vi "ROSSubscriber.vi"(2 "Response":T2, 3 "ROS":T3={"topic port"=1236, "Node"="/labview", "topic"="/robot/head/command_head_nod", "type"="std_msgs/Bool", "node port"=7000, "error "={"status"=FALSE, "code"=0, "source"=""}, "Direction"=enum."Publisher", "Update (ms)"=1, "FIFO size"=1}) -> ()   [LabVIEW 2012]
doc: "Lists nodes with a given topic, requests topics, opens new ports for sunscribers, updates subscribers with master, and closes subscribers"
uses:
  _ROSDefinition.vi
  SubVIs/_ROSDirection.ctl
  SubVIs/_ROSControl.ctl
panel:
  out "publishers":T1(array[cluster])
  out "Queue log":string
  out "read":string
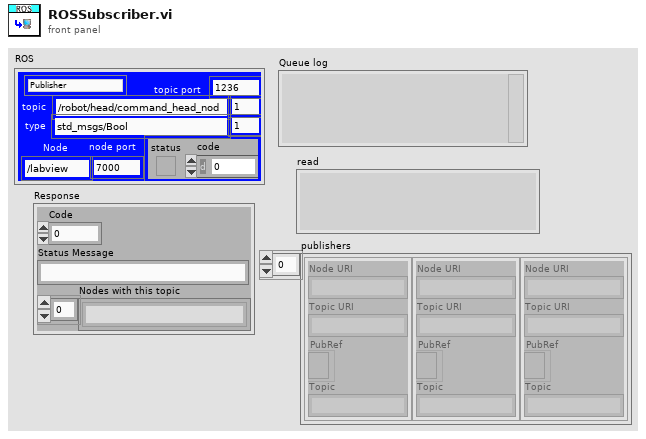
[diagram p1: front panel]
types:
  T1 = cluster{"Node URI":string, "Topic URI":string, "PubRef":refnum<k5>, "Topic":string}[]
  T2 = cluster{"Code":i32, "Status Message":string, "Nodes with this topic":string[]}
  T3 = typedef "_ROSControl.ctl" = cluster{"topic port":u16, "Node":string, "topic":string, "type":string, "node port":u16, "error ":errorcluster, "Direction":T4, "Update (ms)":u16, "FIFO size":u16}
  T4 = typedef "_ROSDirection.ctl" = enum16{"Node", "Publisher", "Subscriber", "ServiceClient", "ServiceProvider"}
  T5 = enum16{"Reset Log", "Add Client", "Remove Client", "Add Task"}
  T6 = cluster{"Node URI":string, "Topic URI":string, "PubRef":refnum<k5>, "Topic":string}
  T7 = cluster{"Caller ID":string, "Topic Name":string, "Node URIs":string[]}
  T8 = cluster{"Protocol":string, "Code":i32, "IP":string, "Port":i32}
  T9 = cluster{"Protocol":string, "Topic URI":string, "PubRef":refnum<k5>, "topic":string}
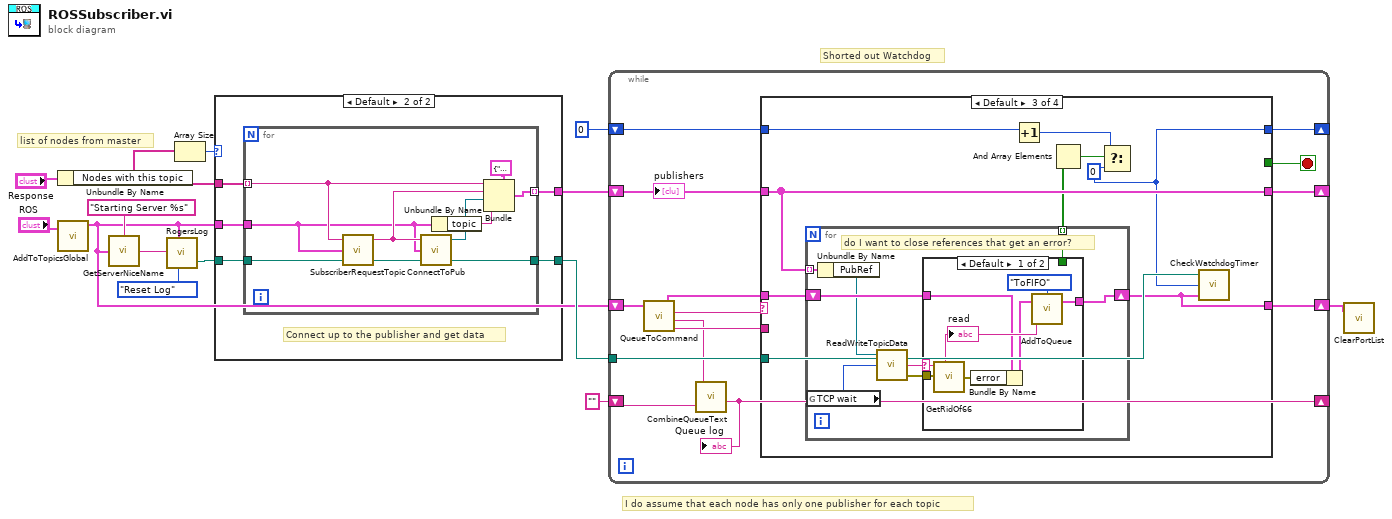
[diagram p0: block diagram]
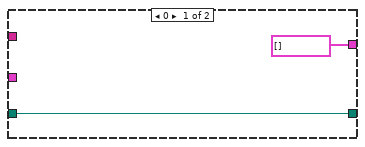
[diagram p2: hidden frame]
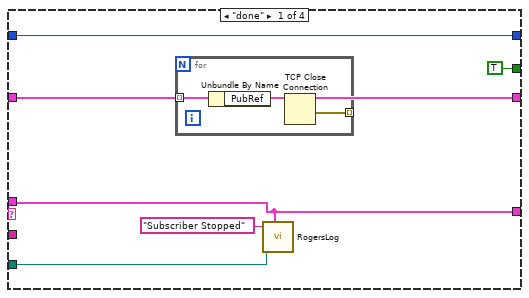
[diagram p3: hidden frame]
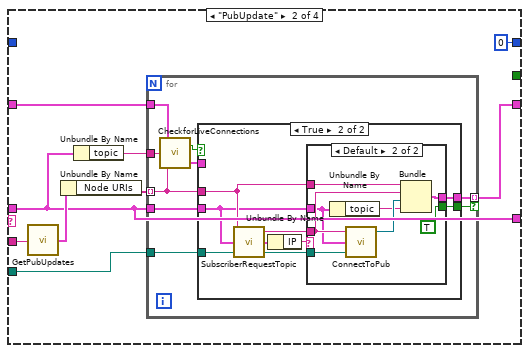
[diagram p4: hidden frame]
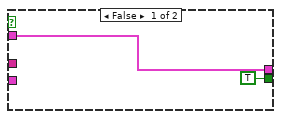
[diagram p5: hidden frame]
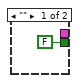
[diagram p6: hidden frame]
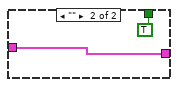
[diagram p7: hidden frame]
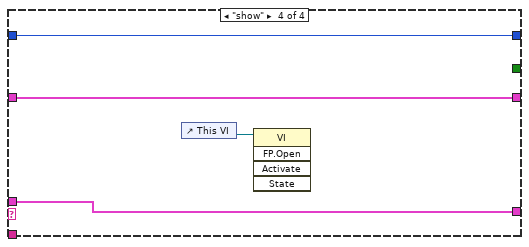
[diagram p8: hidden frame]
diagram:
  # "Shorted out Watchdog"
  # "I do assume that each node has only one publisher for each topic"
  # "list of nodes from master"
  n1 = Unbundle By Name("Response") -> ("Nodes with this topic"=w6:string[])
  n2 = call "AddToTopicsGlobal.vi"("ROS in"="ROS") -> ("ROS out"=w1:T3)  [unwired: 2 in]
  n3 = call "GetServerNiceName.vi"("ROS"=w1, "Text to add"="Starting Server %s") -> ("String"=w11:string)
  n4 = call "RogersLog.vi"("Text to add"=w11, "ROS"=w1, "Task"=T5."Reset Log") -> ("LogPath out"=w9:path)  [unwired: 2 in, 1 out]
  n5 = Array Size(array=w6) -> (size(s)=w5:i32)
  n6 = case shown="Default" w5 {
    tunnel: w6 -> [_ w21]
    tunnel: [T1 [] w20] -> w13
    tunnel: w9 -> [w15 w19]
    tunnel: w1 -> [_ w18]
    tunnel: [w15 w17] -> w8
    frame 0 {
    }
    frame Default {
      # "Connect up to the publisher and get data"
      n7 = for {
        tunnel: w21 -> [w28] mode=indexing
        tunnel: [w25] -> w20 mode=indexing
        tunnel: w19 -> [w31]
        tunnel: w18 -> [w23]
        tunnel: [w29] -> w17
        n8 = call "SubscriberRequestTopic.vi"("LogPath in"=w31, "ROS"=w23, "Node URI"=w28) -> ("LogPath out"=w30:path, "Topic URI"=w27:string)  [unwired: 1 out]
        n9 = call "ConnectToPub.vi"("LogPath in"=w30, "ROS"=w23, "IP"=w27) -> ("LogPath out"=w29:path, "PubRef"=w26:refnum<k5>)  [unwired: 1 out]
        n10 = Unbundle By Name(w23) -> ("topic"=w22:string)
        n11 = Bundle(cluster=T6 {"Node URI"="", "Topic URI"="", "PubRef"=refnum, "Topic"=""} ("output cluster"), "Node URI"=w28, "Topic URI"=w27, "PubRef"=w26, "Topic"=w22) -> (w25:T6)
      }
    }
  }
  n12 = while {
    shift-right: [w41] -> _
    shift-left: w13 -> [w45]
    tunnel: w8 -> [w40]
    shift-right: [w38] -> _
    shift-left: 0 -> [w39]
    shift-right: [w35] -> _
    shift-left: "" ("New List") -> [w37]
    shift-right: [w32] -> w3
    shift-left: w1 -> [w34]
    stop <- w43 stop-if-true
    n13 = call "QueueToCommand.vi"("ROS"=w34) -> ("ROS out"=w33:T3, "Command"=w44:string, "Queue log"=w36:string, "data"=w42:string)  [unwired: 2 in]
    n14 = call "CombineQueueText.vi"("Old List"=w37, "Queue In"=w36) -> ("New List"=w35:string)  [unwired: 1 in]
    "Queue log" <- w35
    n15 = case shown="Default" w44 {
      tunnel: w45 -> [w50 w57 w101 w122]
      tunnel: [TRUE _ _ _] -> w43
      tunnel: w42 -> [_ w61 _ _]
      tunnel: [w50 w58 w101 w122] -> w41
      tunnel: w33 -> [w46 w55 w94 w119]
      tunnel: w40 -> [w48 w59 w96 _]
      tunnel: w39 -> [w47 _ w97 w120]
      tunnel: [w47 0 w95 w120] -> w38
      tunnel: [w46 w55 w93 w119] -> w32
      frame "done" {
        n16 = for {
          tunnel: w50 -> [w53] mode=indexing
          tunnel: [w54] -> _ mode=indexing
          n17 = Unbundle By Name(w53) -> ("PubRef"=w52:refnum<k5>)
          n18 = TCP Close Connection(connection ID=w52) -> (error out=w54:errorcluster)  [unwired: 2 in, 1 out]
        }
        n19 = call "RogersLog.vi"("Text to add"="Subscriber Stopped", "ROS"=w46, "LogPath in"=w48) -> ()  [unwired: 2 in, 2 out]
      }
      frame "PubUpdate" {
        n20 = call "GetPubUpdates.vi"("XML"=w61) -> ("PubUpdate"=w62:T7)
        n21 = Unbundle By Name(w62) -> ("Node URIs"=w60:string[])
        n22 = Unbundle By Name(w55) -> ("topic"=w56:string)
        n23 = for {
          tunnel: w60 -> [w68] mode=indexing
          tunnel: w59 -> [w72]
          tunnel: w55 -> [w71]
          tunnel: [w70] -> w58 mode=indexing if=w64
          tunnel: w57 -> [w69]
          tunnel: w56 -> [w65]
          n24 = call "CheckforLiveConnections.vi"("Node URI"=w68, "topic"=w65, "Connections"=w69) -> ("Connection"=w66:T6, "new?"=w67:bool)
          n25 = case shown="True" w67 {
            tunnel: w72 -> [_ w83]
            tunnel: w71 -> [_ w78]
            tunnel: w68 -> [_ w81]
            tunnel: [w74 w79] -> w70
            tunnel: w66 -> [w74 _]
            tunnel: [TRUE w75] -> w64
            frame False {
            }
            frame True {
              n26 = call "SubscriberRequestTopic.vi"("LogPath in"=w83, "ROS"=w78, "Node URI"=w81) -> ("LogPath out"=w82:path, "Topic Request Reply"=w77:T8, "Topic URI"=w80:string)
              n27 = Unbundle By Name(w77) -> ("IP"=w76:string)
              n28 = case shown="Default" w76 {
                tunnel: w82 -> [_ w92]
                tunnel: w81 -> [_ w91]
                tunnel: w80 -> [_ w90]
                tunnel: [_ w88] -> w79
                tunnel: w78 -> [_ w86]
                tunnel: [FALSE TRUE] -> w75
                frame "" {
                }
                frame Default {
                  n29 = Unbundle By Name(w86) -> ("topic"=w87:string)
                  n30 = call "ConnectToPub.vi"("LogPath in"=w92, "ROS"=w86, "IP"=w90) -> ("PubRef"=w89:refnum<k5>)  [unwired: 2 out]
                  n31 = Bundle("Protocol"=w91, "Topic URI"=w90, "PubRef"=w89, "topic"=w87) -> (w88:T9)  [unwired: 1 in]
                }
              }
            }
          }
        }
      }
      frame Default {
        w95 = 0
        n32 = for {
          tunnel: w101 -> [w105] mode=indexing
          tunnel: [w106] -> w100 mode=indexing
          shift-right: [w103] -> w93
          shift-left: w94 -> [w107]
          # "do I want to close references that get an error?"
          n33 = global read "_ROSDefinition.vi" "TCP wait"() -> (w102:i32)
          n34 = Unbundle By Name(w105) -> ("PubRef"=w104:refnum<k5>)
          n35 = call "ReadWriteTopicData.vi"("timeout ms (1000)"=w102, "connection ID in"=w104) -> ("error out"=w108:errorcluster, "data out"=w109:string)  [unwired: 1 in, 1 out]
          n36 = case shown="Default" w109 {
            selector: w109 -> [w116 _]
            tunnel: w107 -> [w114 w117]
            tunnel: w108 -> [w111 _]
            tunnel: [_ TRUE] -> w106
            tunnel: [w112 w117] -> w103
            frame Default {
              n37 = call "GetRidOf66.vi"("error in (no error)"=w111) -> ("error out"=w110:errorcluster)
              n38 = Bundle By Name(cluster=w114, "error"=w110) -> (w113:T3)
              n39 = call "AddToQueue.vi"("Cmd"=w116, "ROS"=w113, "Type"=enum16{"topic", "node", "ToFIFO"}."ToFIFO") -> ("ROS out"=w112:T3)  [unwired: 2 in]
              "read" <- w116
            }
            frame "" {
            }
          }
        }
        n40 = Increment(x=w97) -> (x+1=w98:i32)
        n41 = And Array Elements(Boolean array=w100) -> (logical AND=w99:bool)
        n42 = Select(t=w98, s=w99, f=w95) -> ()  [unwired: 1 out]
        n43 = call "CheckWatchdogTimer.vi"("ROS"=w93, "itteration"=w95, "LogPath in"=w96) -> ()  [unwired: 3 in]
      }
      frame "show" {
        n44 = control-ref of="This VI"() -> (w121:refnum<vi>)
        n45 = invoke class="VI" method="FP.Open"(reference=w121) -> ()  [unwired: 4 in, 5 out]
      }
    }
    "publishers" <- w45
  }
  n46 = call "ClearPortList.vi"("ROS"=w3) -> ()  [unwired: 2 in]
